vi "Check Channel Number Setting.vi"(1 "Channel Scale Array":fxp<+,24,12>[](array[numeric])=[0.0, 0.0, 0.0, 0.0], 2 "Channel AI Array":fxp<+/-,24,4>[](array[numeric])=[0.0, 0.0, 0.0, 0.0], 3 "Number of Channels":i32) -> (0 "Different Channel Count?":bool)   [LabVIEW 2013]
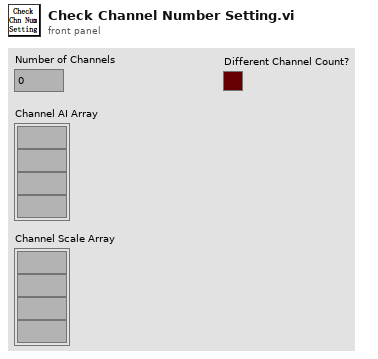
[diagram p1: front panel]
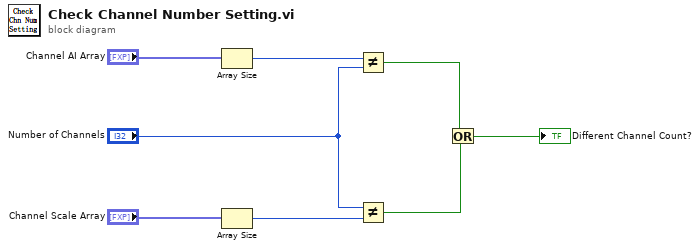
[diagram p0: block diagram]
diagram:
  n1 = Array Size(array="Channel AI Array") -> (size(s)=w7:i32)
  n2 = Array Size(array="Channel Scale Array") -> (size(s)=w4:i32)
  n3 = Not Equal?(x=w7, y="Number of Channels") -> (x != y?=w1:bool)
  n4 = Not Equal?(x="Number of Channels", y=w4) -> (x != y?=w5:bool)
  n5 = Or(x=w1, y=w5) -> (x .or. y?=→"Different Channel Count?":bool)
